vi "PI-C867-JoystickState_Check.vi"(8 "error in (no error)":errorcluster, 11 "State in":bool[][](array[boolean])=[[FALSE], [FALSE], [FALSE], [FALSE], [FALSE], [FALSE]]) -> (0 "error out":errorcluster, 3 "All 0?":bool)   [LabVIEW 2014]
doc: "This VI checks if one button is pressed"
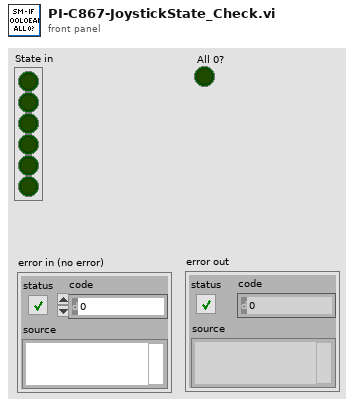
[diagram p1: front panel]
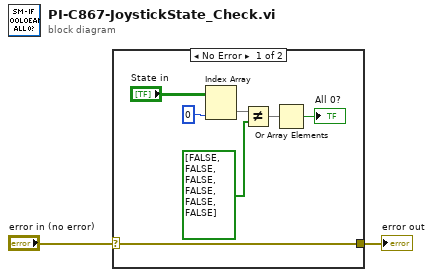
[diagram p0: block diagram]
diagram:
  n1 = case shown="No Error" "error in (no error)" {
    selector: "error in (no error)" -> [w3 w10]
    tunnel: [w3 w10] -> w1
    frame No Error {
      n2 = Index Array(array="State in", index (col)=0 ("disabled index (col)")) -> (element=w6:bool[])  [unwired: 1 in]
      n3 = Not Equal?(x=w6, y=bool[] [FALSE, FALSE, FALSE, FALSE, FALSE, FALSE] ("State")) -> (x != y?=w8:bool[])
      n4 = Or Array Elements(Boolean array=w8) -> (logical OR=→"All 0?":bool)
    }
    frame Error {
    }
  }
  "error out" <- w1
